vi "LoopselFF.VI"() -> ()   [LabVIEW 2015]
uses:
  <vilib>/Analysis/NI_AALBase.lvlib
panel:
  out "variance":dbl
  out "standard deviation":dbl
  out "mean":dbl
  in  "Pixel":u16
  in  "DO8":u16
  in  "TO8":u16
  in  "D02":u16=100
  in  "Send O CTRL":bool
  in  "TM0H":u16
  in  "TM0L":u16=1000
  in  "DO7":u16
  in  "TO7":u16
  in  "DO6":u16
  in  "TO6":u16
  in  "DO5":u16
  in  "TO5":u16
  in  "DO4":u16
  in  "T04":u16
  in  "DO3":u16
  in  "TO3":u16
  in  "TO2":u16=10
  in  "Arm/Clear arry":bool
  in  "Start Read":bool
  in  "?":enum32{"1", "2", "3"}(radio)=enum."3"
  in  "pos slope":u8=1
  in  "both slopes":u8
  in  "DAT in 10ns":u32
  out "FIFO overflow":bool
  in  "extTrig 0/1":u8
  in  "Start Read":bool
  in  "stop all":bool
  in  "Arm/Clear arry":bool
  in  "Slide":u32(slide)=4 scale=1.0..1000.0
  in  "frequency[Hz]":u32
  in  "no.of samples (nos)":u32=100
  in  "exposuretime[ms]":dbl=1.0 format="%.3f"
  out "Signalverlaufgraph":u16[](graph)=[542, 542, 543, 543, 49152, 0, 3, 0, 2, 2, 3, 3, 4, 4, 5, 5, 6, 6, 7, 7, 8, 8, 9, 9, 10, 10, 11, 11, 12, 12, 13, 13, 14, 14, 15, 15, 16, 16, 17, 17, 18, 18, 19, 19, 20, 20, 21, 21, 22, 22, 23, 23, 24, 24, 25, 25, 26, 26, 27, 27, 28, 28, 29, 29, 30, 30, 31, 31, 32, 32, 33, 33, 34, 34, 35, 35, 36, 36, 37, 37, 38, 38, 39, 39, 40, 40, 41, 41, 42, 42, 43, 43, 44, 44, 45, 45, 46, 46, 47, 47, 48, 48, 49, 49, 50, 50, 51, 51, 52, 52, 53, 53, 54, 54, 55, 55, 56, 56, 57, 57, 58, 58, 59, 59, 60, 60, 61, 61, 62, 62, 63, 63, 64, 64, 65, 65, 66, 66, 67, 67, 68, 68, 69, 69, 70, 70, 71, 71, 72, 72, 73, 73, 74, 74, 75, 75, 76, 76, 77, 77, 78, 78, 79, 79, 80, 80, 81, 81, 82, 82, 83, 83, 84, 84, 85, 85, 86, 86, 87, 87, 88, 88, 89, 89, 90, 90, 91, 91, 92, 92, 93, 93, 94, 94, 95, 95, 96, 96, 97, 97, 98, 98, 99, 99, 100, 100, 101, 101, 102, 102, 103, 103, 104, 104, 105, 105, 106, 106, 107, 107, 108, 108, 109, 109, 110, 110, 111, 111, 112, 112, 113, 113, 114, 114, 115, 115, 116, 116, 117, 117, 118, 118, 119, 119, 120, 120, 121, 121, 122, 122, 123, 123, 124, 124, 125, 125, 126, 126, 127, 127, 128, 128, 129, 129, 130, 130, 131, 131, 132, 132, 133, 133, 134, 134, 135, 135, 136, 136, 137, 137, 138, 138, 139, 139, 140, 140, 141, 141, 142, 142, 143, 143, 144, 144, 145, 145, 146, 146, 147, 147, 148, 148, 149, 149, 150, 150, 151, 151, 152, 152, 153, 153, 154, 154, 155, 155, 156, 156, 157, 157, 158, 158, 159, 159, 160, 160, 161, 161, 162, 162, 163, 163, 164, 164, 165, 165, 166, 166, 167, 167, 168, 168, 169, 169, 170, 170, 171, 171, 172, 172, 173, 173, 174, 174, 175, 175, 176, 176, 177, 177, 178, 178, 179, 179, 180, 180, 181, 181, 182, 182, 183, 183, 184, 184, 185, 185, 186, 186, 187, 187, 188, 188, 189, 189, 190, 190, 191, 191, 192, 192, 193, 193, 194, 194, 195, 195, 196, 196, 197, 197, 198, 198, 199, 199, 200, 200, 201, 201, 202, 202, 203, 203, 204, 204, 205, 205, 206, 206, 207, 207, 208, 208, 209, 209, 210, 210, 211, 211, 212, 212, 213, 213, 214, 214, 215, 215, 216, 216, 217, 217, 218, 218, 219, 219, 220, 220, 221, 221, 222, 222, 223, 223, 224, 224, 225, 225, 226, 226, 227, 227, 228, 228, 229, 229, 230, 230, 231, 231, 232, 232, 233, 233, 234, 234, 235, 235, 236, 236, 237, 237, 238, 238, 239, 239, 240, 240, 241, 241, 242, 242, 243, 243, 244, 244, 245, 245, 246, 246, 247, 247, 248, 248, 249, 249, 250, 250, 251, 251, 252, 252, 253, 253, 254, 254, 255, 255, 256, 256, 257, 257, 258, 258, 259, 259, 260, 260, 261, 261, 262, 262, 263, 263, 264, 264, 265, 265, 266, 266, 267, 267, 268, 268, 269, 269, 270, 270, 271, 271, 272, 272, 273, 273, 274, 274, 275, 275, 276, 276, 277, 277, 278, 278, 279, 279, 280, 280, 281, 281, 282, 282, 283, 283, 284, 284, 285, 285, 286, 286, 287, 287, 288, 288, 289, 289, 290, 290, 291, 291, 292, 292, 293, 293, 294, 294, 295, 295, 296, 296, 297, 297, 298, 298, 299, 299, 300, 300, 301, 301, 302, 302, 303, 303, 304, 304, 305, 305, 306, 306, 307, 307, 308, 308, 309, 309, 310, 310, 311, 311, 312, 312, 313, 313, 314, 314, 315, 315, 316, 316, 317, 317, 318, 318, 319, 319, 320, 320, 321, 321, 322, 322, 323, 323, 324, 324, 325, 325, 326, 326, 327, 327, 328, 328, 329, 329, 330, 330, 331, 331, 332, 332, 333, 333, 334, 334, 335, 335, 336, 336, 337, 337, 338, 338, 339, 339, 340, 340, 341, 341, 342, 342, 343, 343, 344, 344, 345, 345, 346, 346, 347, 347, 348, 348, 349, 349, 350, 350, 351, 351, 352, 352, 353, 353, 354, 354, 355, 355, 356, 356, 357, 357, 358, 358, 359, 359, 360, 360, 361, 361, 362, 362, 363, 363, 364, 364, 365, 365, 366, 366, 367, 367, 368, 368, 369, 369, 370, 370, 371, 371, 372, 372, 373, 373, 374, 374, 375, 375, 376, 376, 377, 377, 378, 378, 379, 379, 380, 380, 381, 381, 382, 382, 383, 383, 384, 384, 385, 385, 386, 386, 387, 387, 388, 388, 389, 389, 390, 390, 391, 391, 392, 392, 393, 393, 394, 394, 395, 395, 396, 396, 397, 397, 398, 398, 399, 399, 400, 400, 401, 401, 402, 402, 403, 403, 404, 404, 405, 405, 406, 406, 407, 407, 408, 408, 409, 409, 410, 410, 411, 411, 412, 412, 413, 413, 414, 414, 415, 415, 416, 416, 417, 417, 418, 418, 419, 419, 420, 420, 421, 421, 422, 422, 423, 423, 424, 424, 425, 425, 426, 426, 427, 427, 428, 428, 429, 429, 430, 430, 431, 431, 432, 432, 433, 433, 434, 434, 435, 435, 436, 436, 437, 437, 438, 438, 439, 439, 440, 440, 441, 441, 442, 442, 443, 443, 444, 444, 445, 445, 446, 446, 447, 447, 448, 448, 449, 449, 450, 450, 451, 451, 452, 452, 453, 453, 454, 454, 455, 455, 456, 456, 457, 457, 458, 458, 459, 459, 460, 460, 461, 461, 462, 462, 463, 463, 464, 464, 465, 465, 466, 466, 467, 467, 468, 468, 469, 469, 470, 470, 471, 471, 472, 472, 473, 473, 474, 474, 475, 475, 476, 476, 477, 477, 478, 478, 479, 479, 480, 480, 481, 481, 482, 482, 483, 483, 484, 484, 485, 485, 486, 486, 487, 487, 488, 488, 489, 489, 490, 490, 491, 491, 492, 492, 493, 493, 494, 494, 495, 495, 496, 496, 497, 497, 498, 498, 499, 499, 500, 500, 501, 501, 502, 502, 503, 503, 504, 504, 505, 505, 506, 506, 507, 507, 508, 508, 509, 509, 510, 510, 511, 511, 512, 512, 513, 513, 514, 514, 515, 515, 516, 516, 517, 517, 518, 518, 519, 519, 520, 520, 521, 521, 522, 522, 523, 523, 524, 524, 525, 525, 526, 526, 527, 527, 528, 528, 529, 529, 530, 530, 531, 531, 532, 532, 533, 533, 52860, 52860, 160, 160, 147, 147, 148, 148, 145, 145, 164, 164, 144, 144, 156, 156]
  # "Start with run"
  # "Tn: delay"
  # "Abort with ESC"
  # "Dn: duration"
  # "*5ns"
  # "TO1: T0 main clock"
  # "period"
  # "*10ns"
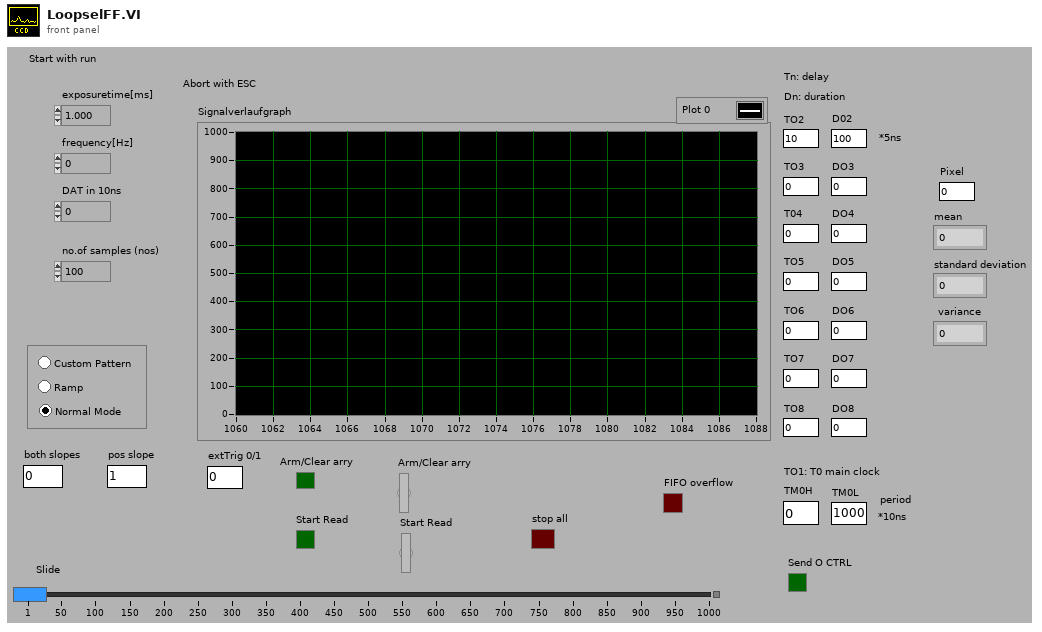
[diagram p1: front panel]
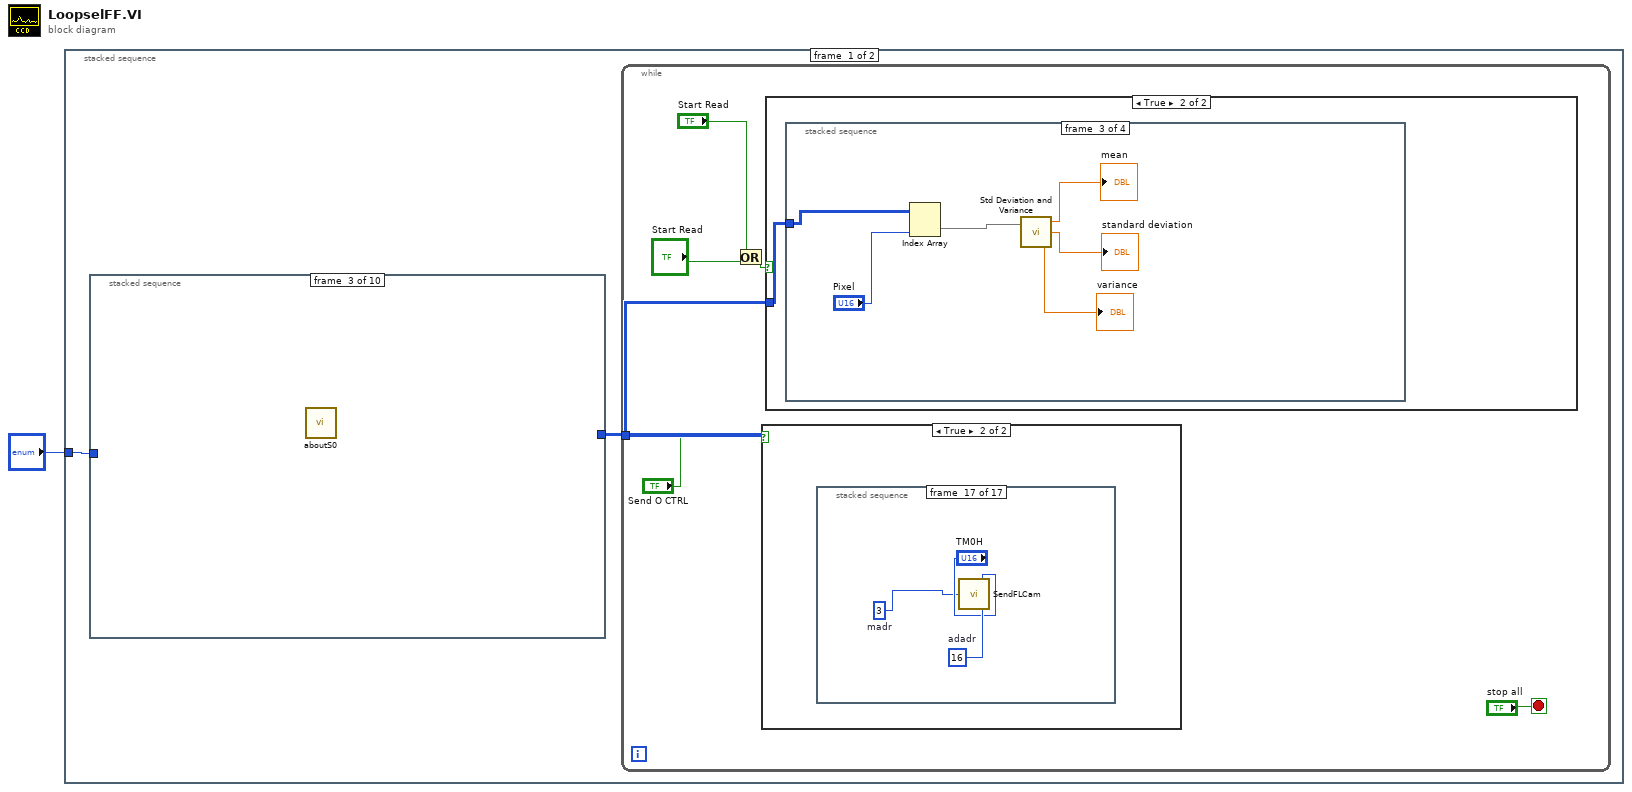
[diagram p0: block diagram]
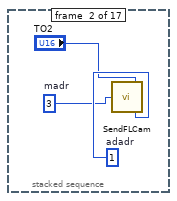
[diagram p4: hidden frame]
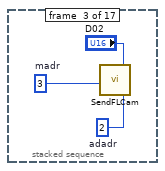
[diagram p5: hidden frame]
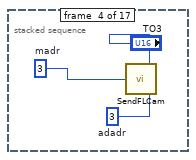
[diagram p6: hidden frame]
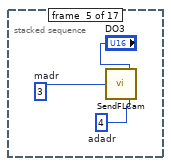
[diagram p7: hidden frame]
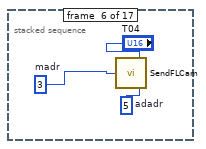
[diagram p8: hidden frame]
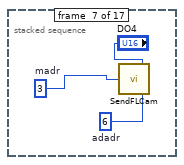
[diagram p9: hidden frame]
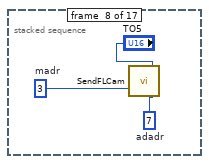
[diagram p10: hidden frame]
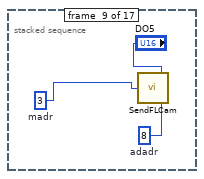
[diagram p11: hidden frame]
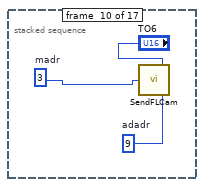
[diagram p12: hidden frame]
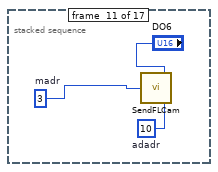
[diagram p13: hidden frame]
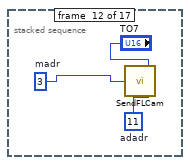
[diagram p14: hidden frame]
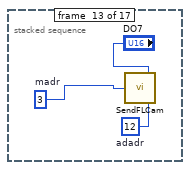
[diagram p15: hidden frame]
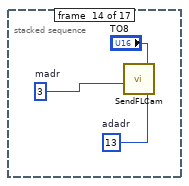
[diagram p16: hidden frame]
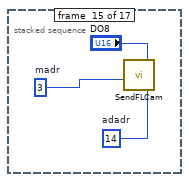
[diagram p17: hidden frame]
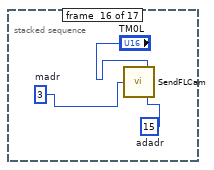
[diagram p18: hidden frame]
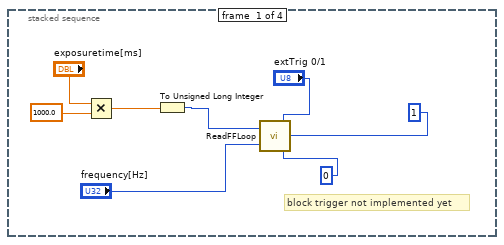
[diagram p20: hidden frame]
diagram:
  n1 = stacked-sequence {
    tunnel: "?" -> [w2 _]
    frame #0 {
      n2 = stacked-sequence {
        tunnel: [_ _ _ _ _ _ _ _ _ w124] -> w3
        tunnel: w2 -> [_ _ _ _ _ w91 _ _ _ _]
        frame #0 {
          n3 = call "InitDrv.vi"() -> ()  [unwired: 1 in]
        }
        frame #1 {
          # "pixel"
          # "xckdelay"
          # "A/D: 2=8bit, 1=12/16bit"
          n4 = call "InitBrd.vi"("xckdly"=u32 0, "pixel"=u32 1088, "flag816"=u32 1) -> ()  [unwired: 3 in]
        }
        frame #2 {
          n5 = call "aboutS0.vi"() -> ()  [unwired: 1 in]
        }
        frame #3 {
          n6 = case shown="1" "both slopes" {
            frame 0, Default {
              n7 = case shown="1" "pos slope" {
                frame 0, Default {
                  n8 = call "LowSlope.vi"() -> ()  [unwired: 1 in]
                }
                frame 1 {
                  n9 = call "HiSlope.vi"() -> ()  [unwired: 1 in]
                }
              }
            }
            frame 1 {
              n10 = call "BothSlopes.vi"() -> ()  [unwired: 1 in]
            }
          }
        }
        frame #4 {
          # "set TrigOut plug to show:"
          # "if (fkt==0)set to XCK -> XCK\nif (fkt==1)set to REG -> OutTrig\nif (fkt==2)set to FFRead\nif (fkt==3)set toTrigIn\nif (fkt==4)set to XCKDLY\nif (fkt==5)set to DAT"
          n11 = call "SetTOREG.vi"("fkt"=u8 0) -> ()
        }
        frame #5 {
          n12 = case shown="\"3\"" w91 {
            frame "1" {
              w92 = 0  # data
              w93 = 38  # adadr
              w94 = 1  # madr
              w95 = 18  # data
              w96 = 37  # adadr
              w97 = 1  # madr
              # "Custom Pattern"
              n13 = call "SendFLCam.vi"("madr"=w97, "data"=w95, "adadr"=w96) -> ()
              n14 = call "SendFLCam.vi"("madr"=w94, "data"=w92, "adadr"=w93) -> ()
            }
            frame "2" {
              w98 = 64  # data
              w99 = 37  # adadr
              w100 = 1  # madr
              # "Ramp"
              n15 = call "SendFLCam.vi"("madr"=w100, "data"=w98, "adadr"=w99) -> ()
            }
            frame "3" {
              w101 = 1  # data
              w103 = 0  # adadr
              w102 = 1  # madr
              w106 = 0  # data
              w105 = 38  # adadr
              w104 = 1  # madr
              w109 = 0  # data
              w108 = 37  # adadr
              w107 = 1  # madr
              # "Normal Mode"
              n16 = call "SendFLCam.vi"("madr"=w104, "data"=w106, "adadr"=w105) -> ()
              n17 = call "SendFLCam.vi"("madr"=w102, "data"=w101, "adadr"=w103) -> ()
              n18 = call "SendFLCam.vi"("madr"=w107, "data"=w109, "adadr"=w108) -> ()
            }
          }
        }
        frame #6 {
          w112 = 5000  # data
          w111 = 1  # adadr
          w110 = 3  # madr
          n19 = call "SendFLCam.vi"("madr"=w110, "data"=w112, "adadr"=w111) -> ()
        }
        frame #7 {
          # "bit31 must be set for enabling DAT(add 0x80000000) to REG 0x20"
          # "is only valid for external trigger!"
          # "this examples shows how to set the DAT (delay after trigger)"
          n20 = Equal To 0?(x="DAT in 10ns") -> (x = 0?=w114:bool)
          n21 = case shown="False" w114 {
            tunnel: "DAT in 10ns" -> [w115 _]
            frame False {
              n22 = Add(x=u32 2147483648, y=w115) -> (x+y=w118:u32)
              n23 = call "WriteL.vi"("val"=w118, "offset"=u32 32) -> ()
            }
            frame True {
              n24 = call "WriteL.vi"("val"=0, "offset"=u32 32) -> ()
            }
          }
        }
        frame #8 {
          # "set gain must be last in init sequence"
          n25 = call "SetAdGain.vi"("gain"=u8 2) -> ()  [unwired: 1 in]
        }
        frame #9 {
          w123 = u32 1088  # PIXEL
          n26 = call "SetupDMA.vi"("pixel"=w123, "nos"="no.of samples (nos)") -> ("Data Values"=w124:u16[][])
        }
      }
      n27 = while {
        tunnel: w3 -> [w9]
        stop <- "stop all" stop-if-true
        n28 = Or(x="Start Read", y="Start Read") -> (x .or. y?=w7:bool)
        n29 = case shown="True" "Send O CTRL" {
          frame False {
          }
          frame True {
            n30 = stacked-sequence {
              frame #0 {
              }
              frame #1 {
                w12 = 1  # adadr
                w11 = 3  # madr
                n31 = call "SendFLCam.vi"("madr"=w11, "data"="TO2", "adadr"=w12) -> ()
              }
              frame #2 {
                w14 = 2  # adadr
                w15 = 3  # madr
                n32 = call "SendFLCam.vi"("madr"=w15, "data"="D02", "adadr"=w14) -> ()
              }
              frame #3 {
                w18 = 3  # adadr
                w17 = 3  # madr
                n33 = call "SendFLCam.vi"("madr"=w17, "data"="TO3", "adadr"=w18) -> ()
              }
              frame #4 {
                w21 = 4  # adadr
                w20 = 3  # madr
                n34 = call "SendFLCam.vi"("madr"=w20, "data"="DO3", "adadr"=w21) -> ()
              }
              frame #5 {
                w24 = 5  # adadr
                w23 = 3  # madr
                n35 = call "SendFLCam.vi"("madr"=w23, "data"="T04", "adadr"=w24) -> ()
              }
              frame #6 {
                w27 = 6  # adadr
                w26 = 3  # madr
                n36 = call "SendFLCam.vi"("madr"=w26, "data"="DO4", "adadr"=w27) -> ()
              }
              frame #7 {
                w30 = 7  # adadr
                w29 = 3  # madr
                n37 = call "SendFLCam.vi"("madr"=w29, "data"="TO5", "adadr"=w30) -> ()
              }
              frame #8 {
                w33 = 8  # adadr
                w32 = 3  # madr
                n38 = call "SendFLCam.vi"("madr"=w32, "data"="DO5", "adadr"=w33) -> ()
              }
              frame #9 {
                w34 = 9  # adadr
                w36 = 3  # madr
                n39 = call "SendFLCam.vi"("madr"=w36, "data"="TO6", "adadr"=w34) -> ()
              }
              frame #10 {
                w39 = 10  # adadr
                w38 = 3  # madr
                n40 = call "SendFLCam.vi"("madr"=w38, "data"="DO6", "adadr"=w39) -> ()
              }
              frame #11 {
                w42 = 11  # adadr
                w41 = 3  # madr
                n41 = call "SendFLCam.vi"("madr"=w41, "data"="TO7", "adadr"=w42) -> ()
              }
              frame #12 {
                w45 = 12  # adadr
                w44 = 3  # madr
                n42 = call "SendFLCam.vi"("madr"=w44, "data"="DO7", "adadr"=w45) -> ()
              }
              frame #13 {
                w47 = 13  # adadr
                w48 = 3  # madr
                n43 = call "SendFLCam.vi"("madr"=w48, "data"="TO8", "adadr"=w47) -> ()
              }
              frame #14 {
                w50 = 14  # adadr
                w51 = 3  # madr
                n44 = call "SendFLCam.vi"("madr"=w51, "data"="DO8", "adadr"=w50) -> ()
              }
              frame #15 {
                w53 = 15  # adadr
                w54 = 3  # madr
                n45 = call "SendFLCam.vi"("madr"=w54, "data"="TM0L", "adadr"=w53) -> ()
              }
              frame #16 {
                w57 = 16  # adadr
                w55 = 3  # madr
                n46 = call "SendFLCam.vi"("madr"=w55, "data"="TM0H", "adadr"=w57) -> ()
              }
            }
          }
        }
        n47 = case shown="True" w7 {
          tunnel: w9 -> [_ w58]
          frame False {
          }
          frame True {
            n48 = stacked-sequence {
              tunnel: w58 -> [_ _ w75 w76]
              frame #0 {
                # "block trigger not implemented yet"
                n49 = Multiply(x="exposuretime[ms]", y=1000.0) -> (x*y=w66:dbl)
                n50 = To Unsigned Long Integer(number=w66) -> (unsigned 32bit integer=w63:u32)
                n51 = call "ReadFFLoop.vi"("exptus"=w63, "freq"="frequency[Hz]", "ExtTrig"="extTrig 0/1", "btrig_ch"=u32 1, "blocktrigger"=u8 0) -> ()
              }
              frame #1 {
                n52 = call "FFOvl.vi"() -> ("FFOvl"=w68:u8)  [unwired: 1 in]
                n53 = Not Equal?(x=w68, y=0) -> (x != y?=→"FIFO overflow":bool)
              }
              frame #2 {
                n54 = Index Array(array=w75, index (col)="Pixel") -> (element=w73:u16[])  [unwired: 1 in]
                n55 = call <vilib>:"Std Deviation and Variance.vi"("X"=w73) -> ("mean"=→"mean":dbl, "standard deviation"=→"standard deviation":dbl, "variance"=→"variance":dbl)  [unwired: 1 in]
              }
              frame #3 {
                n56 = while {
                  tunnel: w76 -> [w78]
                  stop <- w84 continue-if-true
                  n57 = Decrement(x="Slide") -> (x-1=w83:u32)
                  n58 = Index Array(array=w78, index (row)=w83) -> (element=→"Signalverlaufgraph":u16[])  [unwired: 1 in]
                  n59 = Or(x="Arm/Clear arry", y="Arm/Clear arry") -> (x .or. y?=w79:bool)
                  n60 = Not(x=w79) -> (.not. x?=w84:bool)
                }
              }
            }
          }
        }
      }
    }
    frame #1 {
      n61 = call "Exit.vi"() -> ()  [unwired: 1 in]
    }
  }
